vi "Traffic Light.vi"() -> ()   [LabVIEW 2015]
panel:
  out "Green":bool
  out "Yellow":bool
  out "Red":bool
  in  "stop":bool
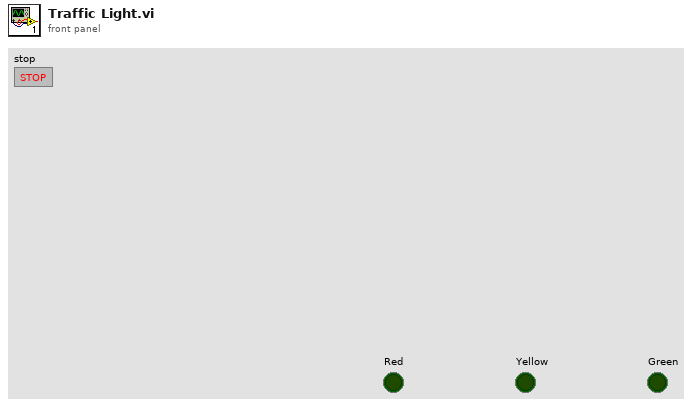
[diagram p1: front panel]
types:
  T1 = enum16{"Red", "Yellow", "Green", "Red and Yellow"}
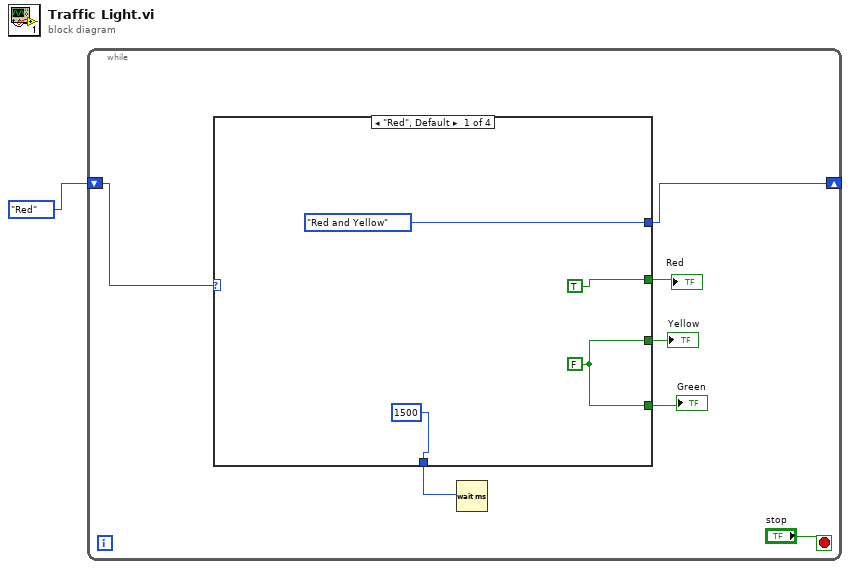
[diagram p0: block diagram]
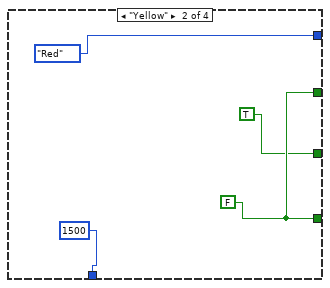
[diagram p2: hidden frame]
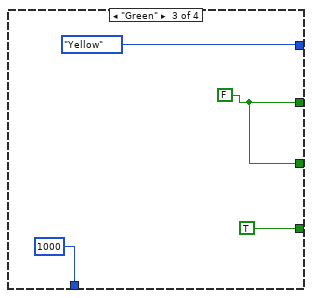
[diagram p3: hidden frame]
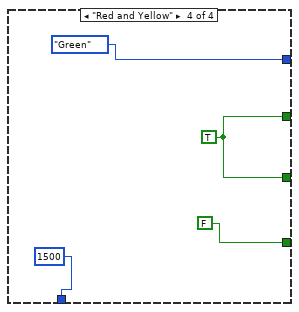
[diagram p4: hidden frame]
diagram:
  n1 = while {
    shift-right: [w7] -> _
    shift-left: T1."Red" -> [w8]
    stop <- "stop" stop-if-true
    n2 = case shown="\"Red\", Default" w8 {
      tunnel: [T1."Red and Yellow" T1."Red" T1."Yellow" T1."Green"] -> w7
      tunnel: [TRUE w15 w19 w23] -> w4
      tunnel: [w10 TRUE w19 w23] -> w5
      tunnel: [w10 w15 TRUE FALSE] -> w3
      tunnel: [1500 1500 u32 1000 ("millisecond timer value") 1500] -> w2
      frame "Red", Default {
        w10 = FALSE
      }
      frame "Yellow" {
        w15 = FALSE
      }
      frame "Green" {
        w19 = FALSE
      }
      frame "Red and Yellow" {
        w23 = TRUE
      }
    }
    "Green" <- w3
    "Red" <- w4
    "Yellow" <- w5
    n3 = Wait (ms)(milliseconds to wait=w2) -> ()  [unwired: 1 out]
  }
